vi "Apply Label Position.vi"(7 "properties to ignore":variant, 8 "error in (no error)":errorcluster, 9 "scaling settings":T1={"scaling factor"={"horizontal"=1.0, "vertical"=1.0}, "scale text"=FALSE} {"scaling factor"."vertical" min=0.0; "scaling factor"."horizontal" min=0.0}, 10 "Ctl Refnum":refnum<vi>, 11 "Control Layout in":refnum<class "Control Layout.lvclass">) -> (0 "error out":errorcluster, 1 "applied?":bool, 3 "Control Layout out":refnum<class "Control Layout.lvclass">)   [LabVIEW 2010, in "NI_SE_Front Panel Layout.lvlib" / "Control Layout.lvclass"]
uses:
  Control Layout.lvclass
  Scaling Factor_Options.ctl
  XY Scaling Factor.ctl
  Object Layout/Object Layout.lvclass/Object Layout.ctl
  Control Layout.lvclass/Control Layout.ctl
  Properties To Ignore.vi
  NI_SE_Front Panel Layout.lvlib
  Object Layout/Object Layout.lvclass
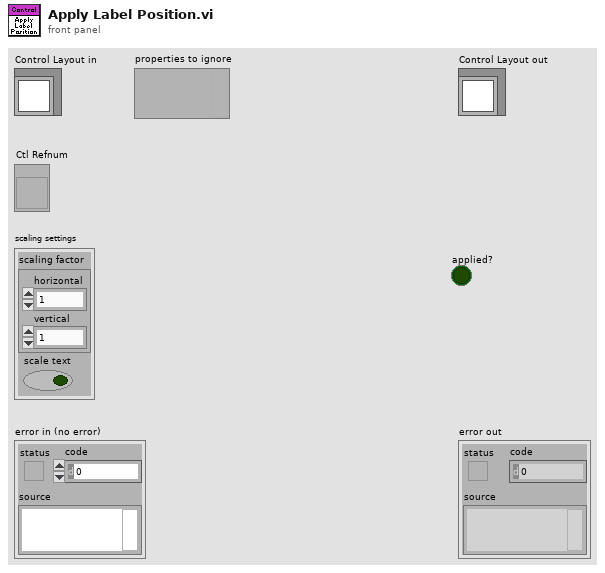
[diagram p1: front panel]
types:
  T1 = typedef "NI_SE_Front Panel Layout.lvlib/Scaling Factor_Options.ctl" = cluster{"scaling factor":T2, "scale text":bool}
  T2 = typedef "NI_SE_Front Panel Layout.lvlib/XY Scaling Factor.ctl" = cluster{"horizontal":dbl, "vertical":dbl}
  T3 = typedef "LVRectTypeDef.ctl" = cluster{"Left":i16, "Top":i16, "Right":i16, "Bottom":i16}
  T4 = typedef "LVPositionTypeDef.ctl" = cluster{"Left":i32, "Top":i32}
  T5 = typedef "LVBoundsTypeDef.ctl" = cluster{"Width":u32, "Height":u32}
  T6 = typedef "LVPointTypeDef.ctl" = cluster{"Horizontal":i16, "Vertical":i16}
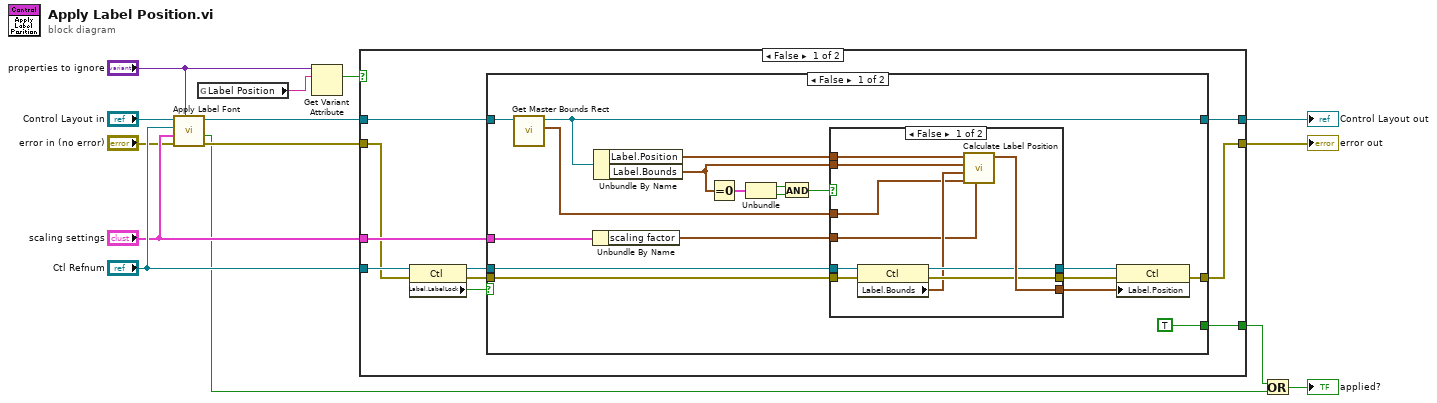
[diagram p0: block diagram]
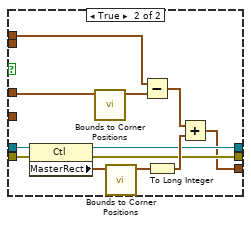
[diagram p2: hidden frame]
diagram:
  n1 = call "Apply Label Font.vi"("properties to ignore"="properties to ignore", "error in (no error)"="error in (no error)", "scaling settings"="scaling settings", "Ctl Refnum"="Ctl Refnum", "Control Layout in"="Control Layout in") -> ("error out"=w4:errorcluster, "applied?"=w3:bool, "Control Layout out"=w9:refnum<class "Control Layout.lvclass">)  [unwired: 4 in]
  n2 = global read "Properties To Ignore.vi" "Label Position"() -> (w11:string)
  n3 = Get Variant Attribute(Variant="properties to ignore", name=w11) -> (found=w12:bool)  [unwired: 2 in, 3 out]
  n4 = case shown="False" w12 {
    tunnel: w4 -> [w17 w67]
    tunnel: [w24 w67] -> w14
    tunnel: w9 -> [w21 w68]
    tunnel: "scaling settings" -> [w23 _]
    tunnel: "Ctl Refnum" -> [w19 _]
    tunnel: [w20 w68] -> w13
    tunnel: [w22 _] -> w1
    frame False {
      n5 = property class="Ctl"(reference=w19, error in=w17) -> (reference out=w18:refnum<vi>, error out=w16:errorcluster, "Label.LabelLock"=w15:bool)
      n6 = case shown="False" w15 {
        tunnel: [w42 w65] -> w24
        tunnel: w23 -> [w41 _]
        tunnel: [TRUE _] -> w22
        tunnel: w21 -> [w38 w66]
        tunnel: [w37 w66] -> w20
        tunnel: w18 -> [w31 _]
        tunnel: w16 -> [w30 w65]
        frame False {
          n7 = call "Get Master Bounds Rect.vi"("Object Layout in"=w38) -> ("Rect"=w36:T3, "Object Layout out"=w37:refnum<class "Control Layout.lvclass">)  [unwired: 8 in, 1 out]
          n8 = Unbundle By Name(w41) -> ("scaling factor"=w40:T2)
          n9 = Unbundle By Name(w37) -> ("Label.Position"=w35:T4, "Label.Bounds"=w29:T5)
          n10 = Equal To 0?(x=w29) -> (x = 0?=w28:cluster{"Width":bool, "Height":bool})
          n11 = Unbundle(w28) -> ("Width"=w27:bool, "Height"=w26:bool)
          n12 = And(x=w27, y=w26) -> (x .and. y?=w25:bool)
          n13 = case shown="False" w25 {
            tunnel: w35 -> [w52 w56]
            tunnel: [w51 w57] -> w32
            tunnel: w40 -> [w43 _]
            tunnel: w29 -> [w50 _]
            tunnel: w31 -> [w49 w61]
            tunnel: [w48 w58] -> w34
            tunnel: w30 -> [w47 w60]
            tunnel: [w46 w59] -> w33
            tunnel: w36 -> [w44 w54]
            frame False {
              n14 = property class="Ctl"(reference=w49, error in=w47) -> (reference out=w48:refnum<vi>, error out=w46:errorcluster, "Label.Bounds"=w45:T5)
              n15 = call "Calculate Label Position.vi"("scaling factor"=w43, "layout owner bounds"=w44, "scaled object size"=w45, "layout object size"=w50, "layout label position"=w52) -> ("scaled label position"=w51:T4)  [unwired: 6 in]
            }
            frame True {
              n16 = property class="Ctl"(reference=w61, error in=w60) -> (reference out=w58:refnum<vi>, error out=w59:errorcluster, "MasterRect"=w64:T3)
              n17 = call "Bounds to Corner Positions.vi"("bounds"=w54) -> ("top left"=w53:T6)  [unwired: 9 in, 1 out]
              n18 = call "Bounds to Corner Positions.vi"("bounds"=w64) -> ("top left"=w63:T6)  [unwired: 9 in, 1 out]
              n19 = Subtract(x=w56, y=w53) -> (x-y=w55:T4)
              n20 = To Long Integer(number=w63) -> (32bit integer=w62:cluster{"Horizontal":i32, "Vertical":i32})
              n21 = Add(x=w55, y=w62) -> (x+y=w57:T4)
            }
          }
          n22 = property class="Ctl"(reference=w34, error in=w33, "Label.Position"=w32) -> (error out=w42:errorcluster)  [unwired: 1 out]
        }
        frame True {
        }
      }
    }
    frame True {
    }
  }
  "error out" <- w14
  "Control Layout out" <- w13
  n23 = Or(x=w1, y=w3) -> (x .or. y?=→"applied?":bool)
